vi "콜라자판기.vi"() -> ()   [LabVIEW 2014]
panel:
  out "링":u16(ring)
  in  "종료":bool
  in  "반환":bool
  in  "구매":bool
  out "투입금액":i32
  in  "동전":T1
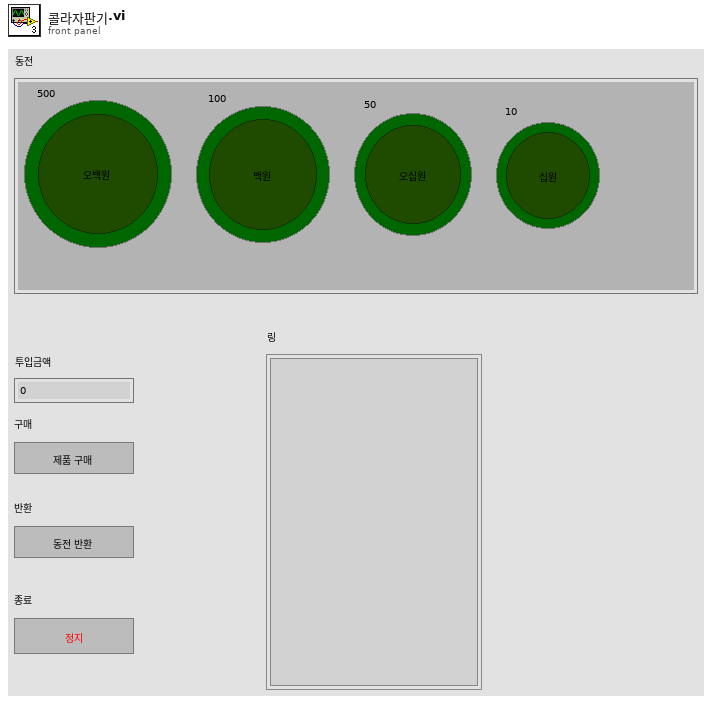
[diagram p1: front panel]
types:
  T1 = cluster{"500":bool, "100":bool, "50":bool, "10":bool}
  T2 = enum8{"Enabled", "Disabled", "Disabled and Grayed Out"}
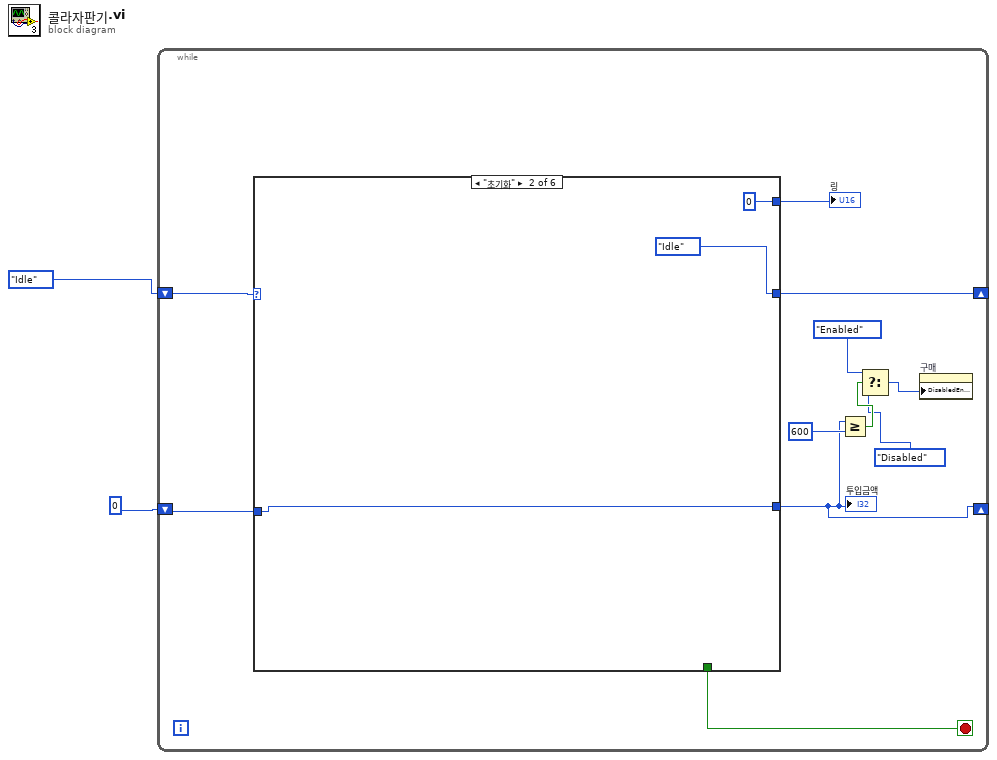
[diagram p0: block diagram]
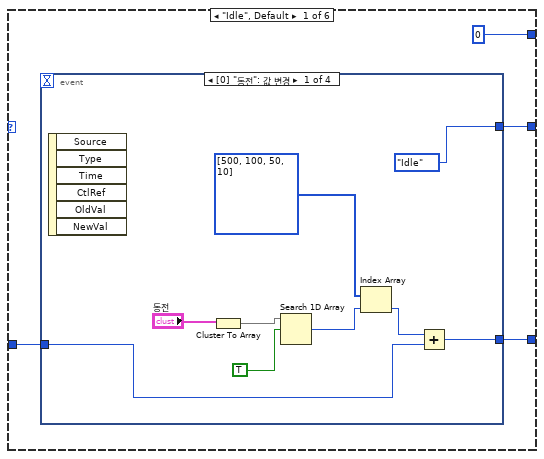
[diagram p2: hidden frame]
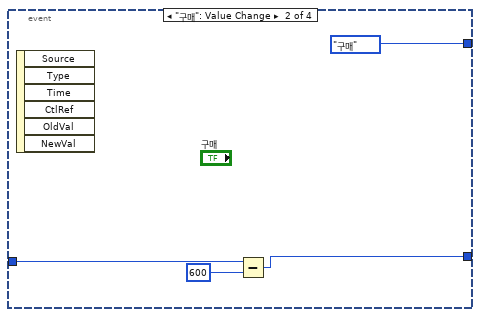
[diagram p3: hidden frame]
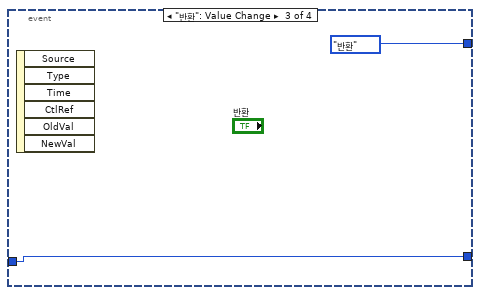
[diagram p4: hidden frame]
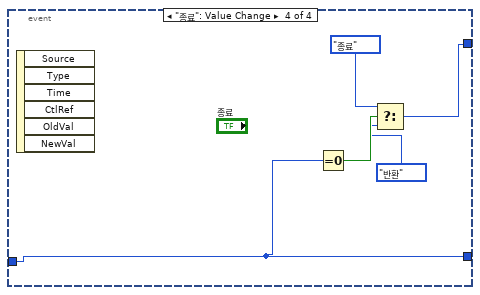
[diagram p5: hidden frame]
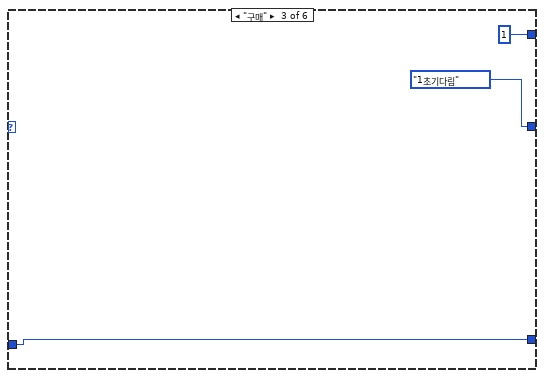
[diagram p6: hidden frame]
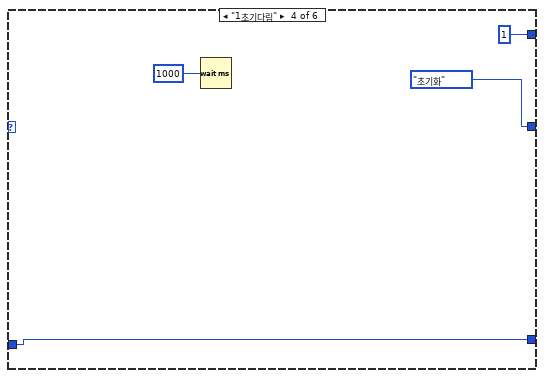
[diagram p7: hidden frame]
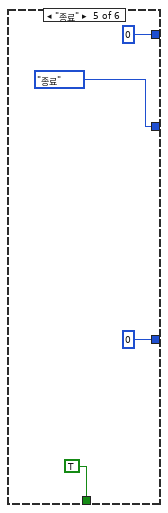
[diagram p8: hidden frame]
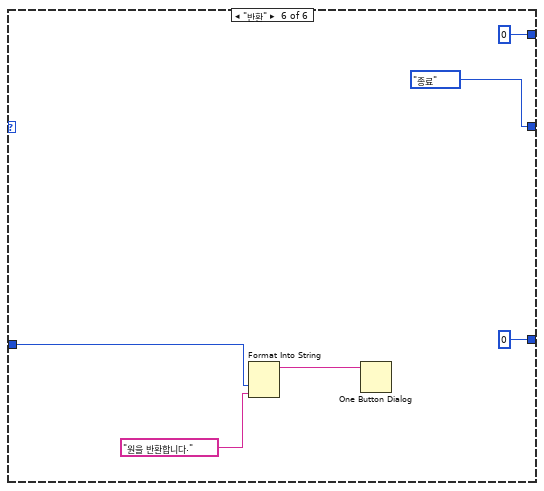
[diagram p9: hidden frame]
diagram:
  n1 = while {
    shift-right: [w12] -> _
    shift-left: enum16{"Idle", "초기화", "종료", "구매", "반환", "1초기다림"}."Idle" ("열거형") -> [w13]
    shift-right: [w8] -> _
    shift-left: 0 -> [w11]
    stop <- w3 stop-if-true
    n2 = case shown="\"초기화\"" w13 {
      tunnel: [w17 enum16{"Idle", "초기화", "종료", "구매", "반환", "1초기다림"}."Idle" ("열거형") enum16{"Idle", "초기화", "종료", "구매", "반환", "1초기다림"}."1초기다림" ("열거형") enum16{"Idle", "초기화", "종료", "구매", "반환", "1초기다림"}."초기화" ("열거형") enum16{"Idle", "초기화", "종료", "구매", "반환", "1초기다림"}."종료" ("열거형") enum16{"Idle", "초기화", "종료", "구매", "반환", "1초기다림"}."종료" ("열거형")] -> w12
      tunnel: w11 -> [w16 w38 w41 w45 _ w54]
      tunnel: [u16 0 u16 0 u16 1 u16 1 u16 0 u16 0] -> w10
      tunnel: [w14 w38 w41 w45 0 0] -> w8
      tunnel: [_ _ _ _ TRUE _] -> w3
      frame "Idle", Default {
        n3 = event shown="[0] \"동전\": 값 변경" {
          selector: _ -> [_ _ _ _]
          dyn-events: _ -> [_ _ _ _]
          timeout: _ -> [_ _ _ _]
          tunnel: [enum16{"Idle", "초기화", "종료", "구매", "반환", "1초기다림"}."Idle" ("열거형") enum16{"Idle", "초기화", "종료", "구매", "반환", "1초기다림"}."구매" ("열거형") enum16{"Idle", "초기화", "종료", "구매", "반환", "1초기다림"}."반환" ("열거형") w35] -> w17
          tunnel: w16 -> [w18 w29 w31 w37]
          tunnel: [w19 w28 w31 w37] -> w14
          event "동전": Value Change {
            n4 = event-data() -> ()  [unwired: 1 in, 6 out]
            n5 = Cluster To Array(cluster="동전") -> (array=w24:bool[])
            n6 = Search 1D Array(1D array=w24, element=TRUE) -> (index of element=w21:i32)  [unwired: 1 in]
            n7 = Index Array(array=i32[] [500, 100, 50, 10], index=w21) -> (element=w20:i32)
            n8 = Add(x=w20, y=w18) -> (x+y=w19:i32)
          }
          event "구매": Value Change {
            n9 = event-data() -> ()  [unwired: 1 in, 6 out]
            n10 = Subtract(x=w29, y=600) -> (x-y=w28:i32)
          }
          event "반환": Value Change {
            n11 = event-data() -> ()  [unwired: 1 in, 6 out]
          }
          event "종료": Value Change {
            n12 = event-data() -> ()  [unwired: 1 in, 6 out]
            n13 = Equal To 0?(x=w37) -> (x = 0?=w36:bool)
            n14 = Select(t=enum16{"Idle", "초기화", "종료", "구매", "반환", "1초기다림"}."종료" ("열거형"), s=w36, f=enum16{"Idle", "초기화", "종료", "구매", "반환", "1초기다림"}."반환" ("열거형")) -> (s? t:f=w35:enum16{"Idle", "초기화", "종료", "구매", "반환", "1초기다림"})
          }
        }
      }
      frame "초기화" {
      }
      frame "구매" {
      }
      frame "1초기다림" {
        n15 = Wait (ms)(milliseconds to wait=u32 1000 ("대기 시간(ms)")) -> ()  [unwired: 1 out]
      }
      frame "종료" {
      }
      frame "반환" {
        n16 = Format Into String(w54, "원을 반환합니다.") -> (resulting string=w52:string)  [unwired: 3 in, 1 out]
        n17 = One Button Dialog(message=w52) -> ()  [unwired: 1 in, 1 out]
      }
    }
    "링" <- w10
    "투입금액" <- w8
    n18 = Greater Or Equal?(x=w8, y=600) -> (x >= y?=w7:bool)
    n19 = Select(t=T2."Enabled" ("비활성화"), s=w7, f=T2."Disabled" ("비활성화")) -> (s? t:f=w5:T2)
    n20 = property on="구매" class="Bool"("DisabledEnum"=w5) -> ()  [unwired: 2 in, 2 out]
  }
